vi "Servo1.vi"() -> ()   [LabVIEW 2023]
uses:
  <vilib>/MakerHub/LINX/Public/Utilities/Open Serial.vi
  <vilib>/MakerHub/LINX/Public/Sensors/Motion/Servo/Servo Open One Channel.vi
  <vilib>/MakerHub/LINX/Public/Sensors/Motion/Servo/Servo Set Pulse Width One Channel.vi
  <vilib>/MakerHub/LINX/Public/Sensors/Motion/Servo/Servo Close One Channel.vi
  <vilib>/MakerHub/LINX/LMH-LINX.lvlib
  <vilib>/MakerHub/LINX/Public/Sensors/Motion/Servo/Servo.lvlib
panel:
  in  "Serial Port":refnum<visa-resource-name>="N/A"
  in  "Servo 2":dbl(knob) scale=500.0..2400.0
  in  "Servo 1":dbl(knob) scale=500.0..2400.0
  in  "Reset":bool
  in  "stop":bool
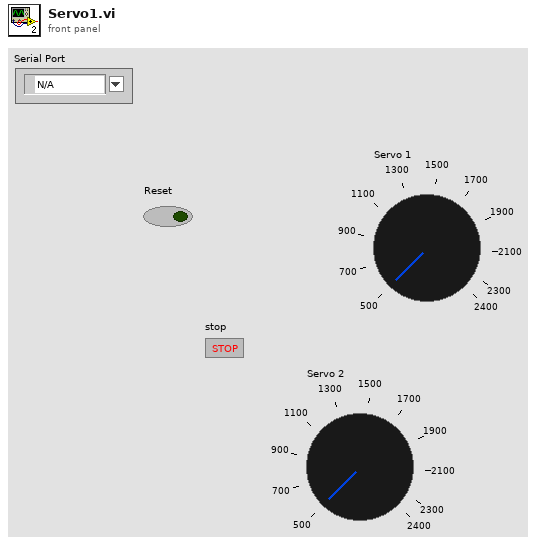
[diagram p1: front panel]
types:
  T1 = typedef "LMH-LINX.lvlib/LINX Ref.ctl" = cluster{"IO":T2, "Interface":T3, "LINX Device Config":T4}
  T2 = typedef "LMH-LINX.lvlib/Platform.ctl" = enum16{"Remote", "Local"}
  T3 = typedef "LMH-LINX.lvlib/Interface.ctl" = enum16{"Serial", "TCP"}
  T4 = typedef "LMH-LINX.lvlib/Device.lvlib/LINX Device Config.ctl" = cluster{"Interface":T3, "COM Port":refnum<visa-resource-name>, "TCP Configuration":T5, "Device Family":u8, "Device ID":u8, "Device Name":string, "TCP Ref":refnum<k5>, "Channels":T6}
  T5 = typedef "LMH-LINX.lvlib/Device.lvlib/TCP Config.ctl" = cluster{"IP Address":string, "Port":u16}
  T6 = typedef "LMH-LINX.lvlib/Channels.ctl" = cluster{"DI":u8[], "DO":u8[], "AI":u8[], "AO":u8[], "PWM":u8[], "QE":u8[], "UART":u8[], "I2C 2":u8[], "SPI":u8[], "CAN":u8[], "Servo":u8[], "AI Ref (V)":dbl, "AI Resolution (Bits)":u8, "AO Ref (V)":dbl, "AO Resolution (Bits)":u8}
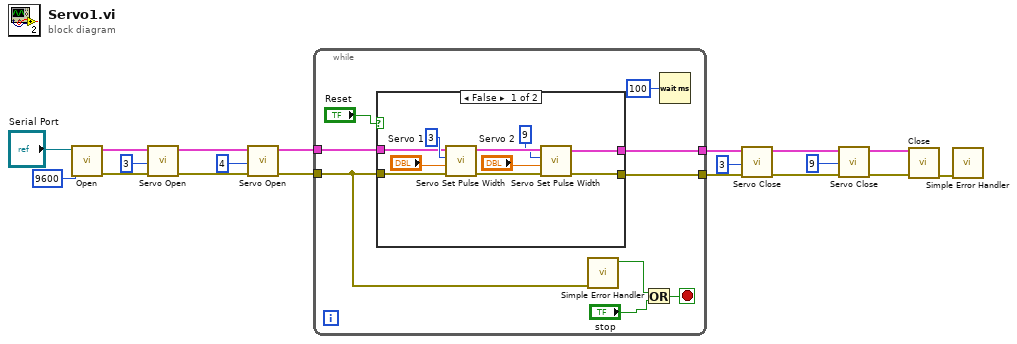
[diagram p0: block diagram]
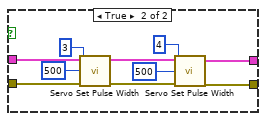
[diagram p2: hidden frame]
diagram:
  n1 = call-poly <vilib>:"Open.vi"("Baud Rate Override"=u32 9600, "Serial Port"="Serial Port") -> ("Error Out"=w19:errorcluster, "LINX Resource"=w18:T1)  [unwired: 7 in, 1 out]
  n2 = call-poly <vilib>:"Servo Open.vi"("Error In"=w19, "Servo Channel"=u8 3, "LINX Resource"=w18) -> ("Error Out"=w17:errorcluster, "LINX Resource"=w16:T1)  [unwired: 7 in]
  n3 = call-poly <vilib>:"Servo Open.vi"("Error In"=w17, "Servo Channel"=u8 4, "LINX Resource"=w16) -> ("Error Out"=w3:errorcluster, "LINX Resource"=w4:T1)  [unwired: 7 in]
  n4 = while {
    tunnel: [w28] -> w9
    tunnel: [w27] -> w8
    tunnel: w4 -> [w23]
    tunnel: w3 -> [w21]
    stop <- w26 stop-if-true
    n5 = case shown="False" "Reset" {
      tunnel: [w31 w48] -> w28
      tunnel: [w32 w47] -> w27
      tunnel: w23 -> [w34 w44]
      tunnel: w21 -> [w33 w41]
      frame False {
        n6 = call-poly <vilib>:"Servo Set Pulse Width.vi"("Error In"=w33, "Pulse Width (uS)"="Servo 1", "Servo Channel"=u8 3, "LINX Resource"=w34) -> ("Error Out"=w38:errorcluster, "LINX Resource"=w37:T1)  [unwired: 6 in]
        n7 = call-poly <vilib>:"Servo Set Pulse Width.vi"("Error In"=w38, "Pulse Width (uS)"="Servo 2", "Servo Channel"=u8 9, "LINX Resource"=w37) -> ("Error Out"=w32:errorcluster, "LINX Resource"=w31:T1)  [unwired: 6 in]
      }
      frame True {
        n8 = call-poly <vilib>:"Servo Set Pulse Width.vi"("Error In"=w41, "Pulse Width (uS)"=u16 500, "Servo Channel"=u8 3, "LINX Resource"=w44) -> ("Error Out"=w45:errorcluster, "LINX Resource"=w46:T1)  [unwired: 6 in]
        n9 = call-poly <vilib>:"Servo Set Pulse Width.vi"("Error In"=w45, "Pulse Width (uS)"=u16 500, "Servo Channel"=u8 4, "LINX Resource"=w46) -> ("Error Out"=w47:errorcluster, "LINX Resource"=w48:T1)  [unwired: 6 in]
      }
    }
    n10 = call <vilib>:"Simple Error Handler.vi"("error in (no error)"=w21) -> ("error?"=w25:bool)  [unwired: 4 in, 4 out]
    n11 = Or(x=w25, y="stop") -> (x .or. y?=w26:bool)
    n12 = Wait (ms)(milliseconds to wait=u32 100) -> ()  [unwired: 1 out]
  }
  n13 = call-poly <vilib>:"Servo Close.vi"("Error In"=w8, "Servo Channel"=u8 3, "LINX Resource"=w9) -> ("Error Out"=w11:errorcluster, "LINX Resource"=w10:T1)  [unwired: 7 in]
  n14 = call-poly <vilib>:"Servo Close.vi"("Error In"=w11, "Servo Channel"=u8 9, "LINX Resource"=w10) -> ("Error Out"=w13:errorcluster, "LINX Resource"=w12:T1)  [unwired: 7 in]
  n15 = call <vilib>:"Close.vi"("Error In"=w13, "LINX Resource"=w12) -> ("Error Out"=w5:errorcluster)  [unwired: 9 in]
  n16 = call <vilib>:"Simple Error Handler.vi"("error in (no error)"=w5) -> ()  [unwired: 4 in, 5 out]
